vi "IB_RW_Project_MSI.vi"(7 "action":T1, 8 "error in (no error)":errorcluster, 9 "ProjectPath":path, 10 "MSI in":T2={"upgradeCode"="", "distID"="", "windowMessage"="", "windowTitle"="", "arpPhone"="", "arpContact"="", "arpURL"="http://", "arpCompany"="", "licenseID"="", "welcomeImageID"="", "bannerImageID"="", "osCheck"=0, "msiFileName"="", "cabFileName"="", "hwOption"=enum."<none>", "hwPath"=path "", "winsec.certificate"="", "winsec.timestamp"="", "winsec.description"="", "autoselect drivers"=FALSE, "hide non-runtimes"=FALSE}, 11 "Object In":T4) -> (0 "error out":errorcluster, 2 "MSI out":T2={"upgradeCode"="", "distID"="", "windowMessage"="", "windowTitle"="", "arpPhone"="", "arpContact"="", "arpURL"="http://", "arpCompany"="", "licenseID"="", "welcomeImageID"="", "bannerImageID"="", "osCheck"=0, "msiFileName"="", "cabFileName"="", "hwOption"=enum."<none>", "hwPath"=path "", "winsec.certificate"="", "winsec.timestamp"="", "winsec.description"="", "autoselect drivers"=FALSE, "hide non-runtimes"=FALSE}, 3 "Object Out":T4)   [LabVIEW 2020]
uses:
  <vilib>/AppBuilder/AB_Relative_Path_Type.ctl
  <resource>/Framework/Providers/API/ItemRef.ctl
  <resource>/Framework/Providers/Builds/Installer/CDK_sTypeDef_HWImportOption.ctl
  <vilib>/AppBuilder/IB_RW_Project/IB_RW_Project_MSI_Data.ctl
  <vilib>/AppBuilder/IB_RW_Project/IB_RW_Project_PropBag_Action.ctl
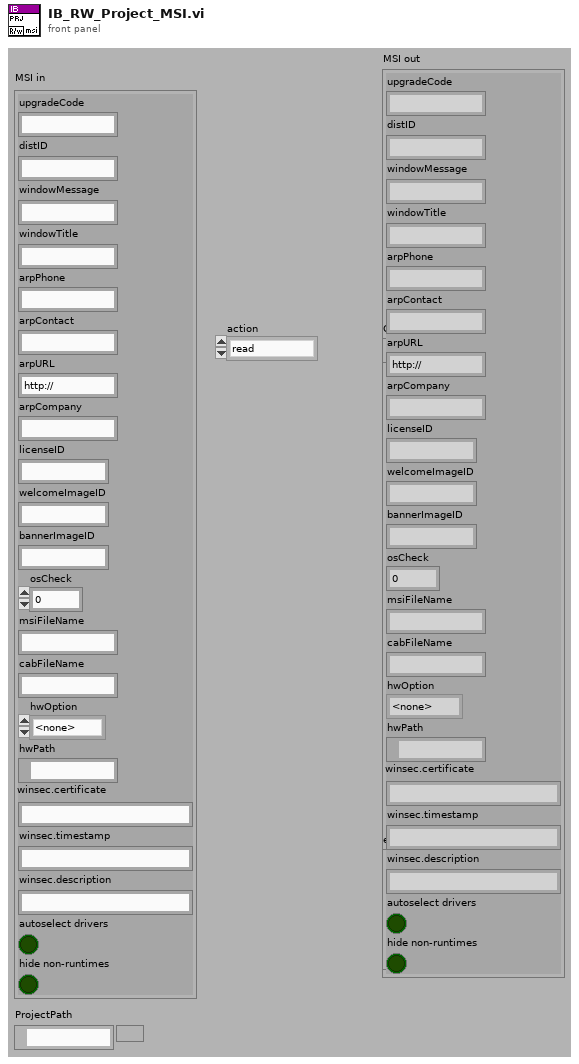
[diagram p1: front panel]
types:
  T1 = typedef "IB_RW_Project_PropBag_Action.ctl" = enum16{"read", "write", "clear", "readPrevious", "writePrevious", "clearPrevious"}
  T2 = typedef "IB_RW_Project_MSI_Data.ctl" = cluster{"upgradeCode":string, "distID":string, "windowMessage":string, "windowTitle":string, "arpPhone":string, "arpContact":string, "arpURL":string, "arpCompany":string, "licenseID":string, "welcomeImageID":string, "bannerImageID":string, "osCheck":i32, "msiFileName":string, "cabFileName":string, "hwOption":T3, "hwPath":path, "winsec.certificate":string, "winsec.timestamp":string, "winsec.description":string, "autoselect drivers":bool, "hide non-runtimes":bool}
  T3 = typedef "CDK_sTypeDef_HWImportOption.ctl" = enum16{"<none>", "Merge", "Replace", "Dialog"}
  T4 = typedef "ItemRef.ctl" = u64
  T5 = typedef "AB_Relative_Path_Type.ctl" = enum16{"<none>", "relativeToCommon", "relativeToAppDir", "relativeToProject"}
  T6 = typedef "IB_Relative_Path_Type.ctl" = enum16{"<none>", "relativeToCommon", "relativeToAppDir", "relativeToProject"}
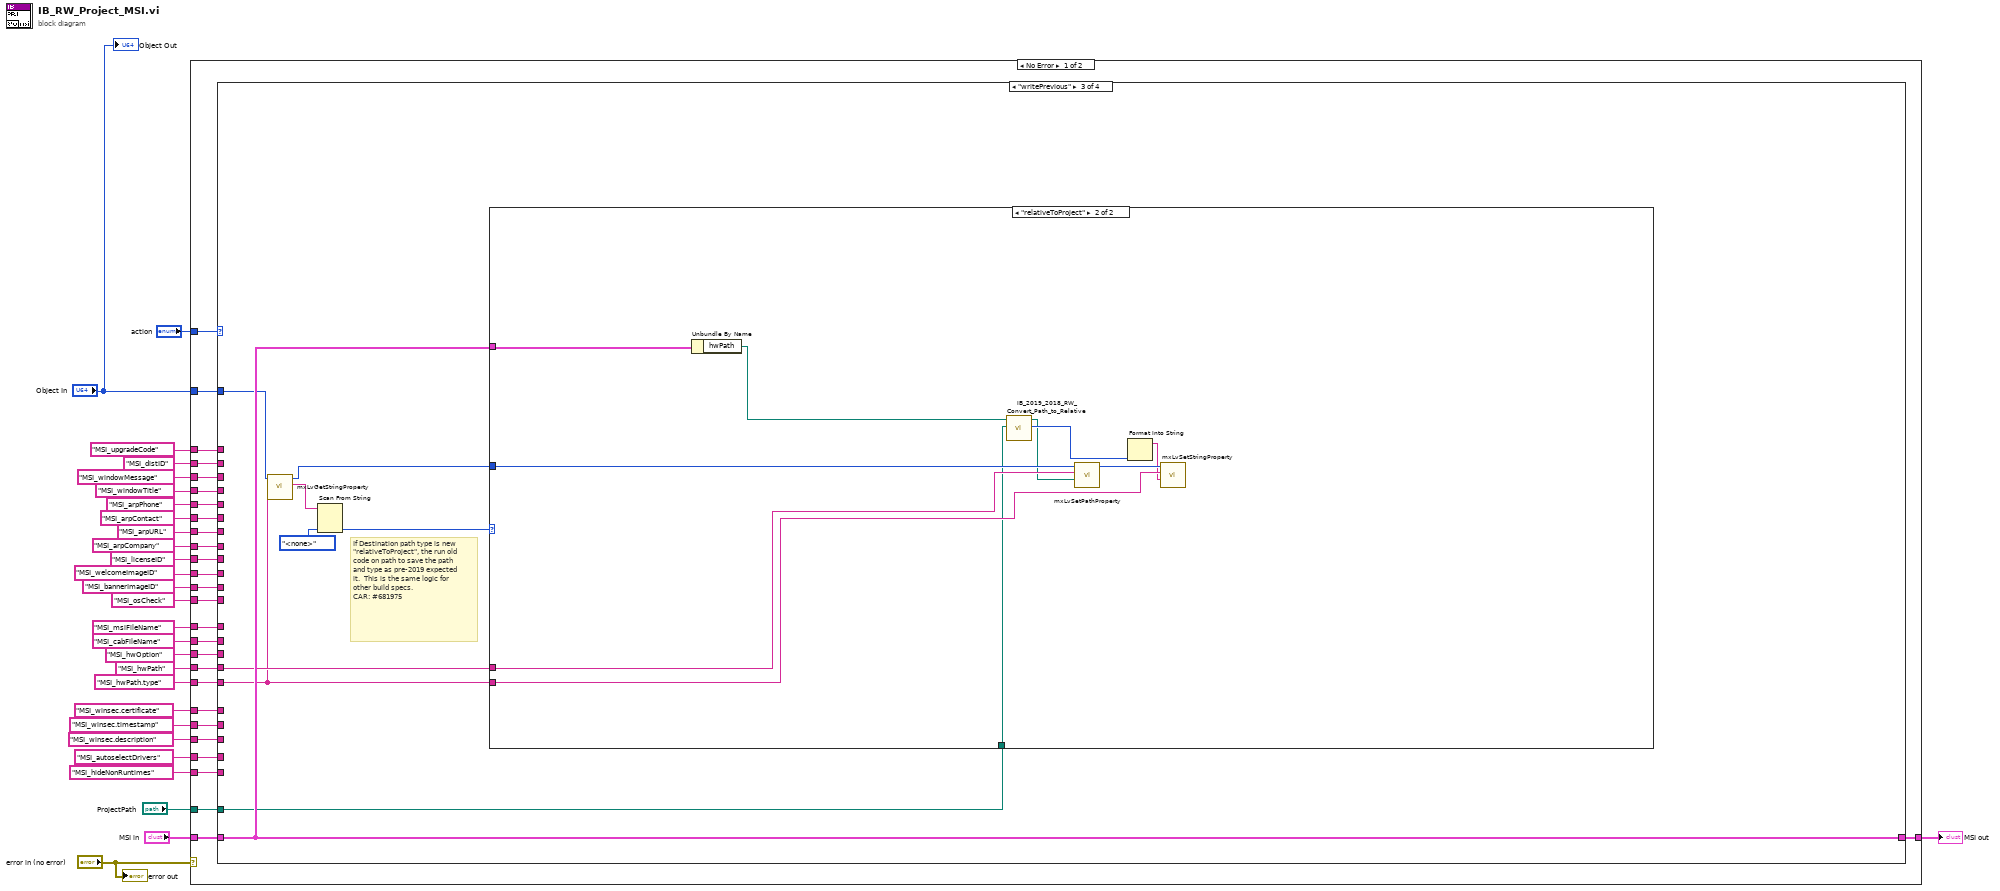
[diagram p0: block diagram]
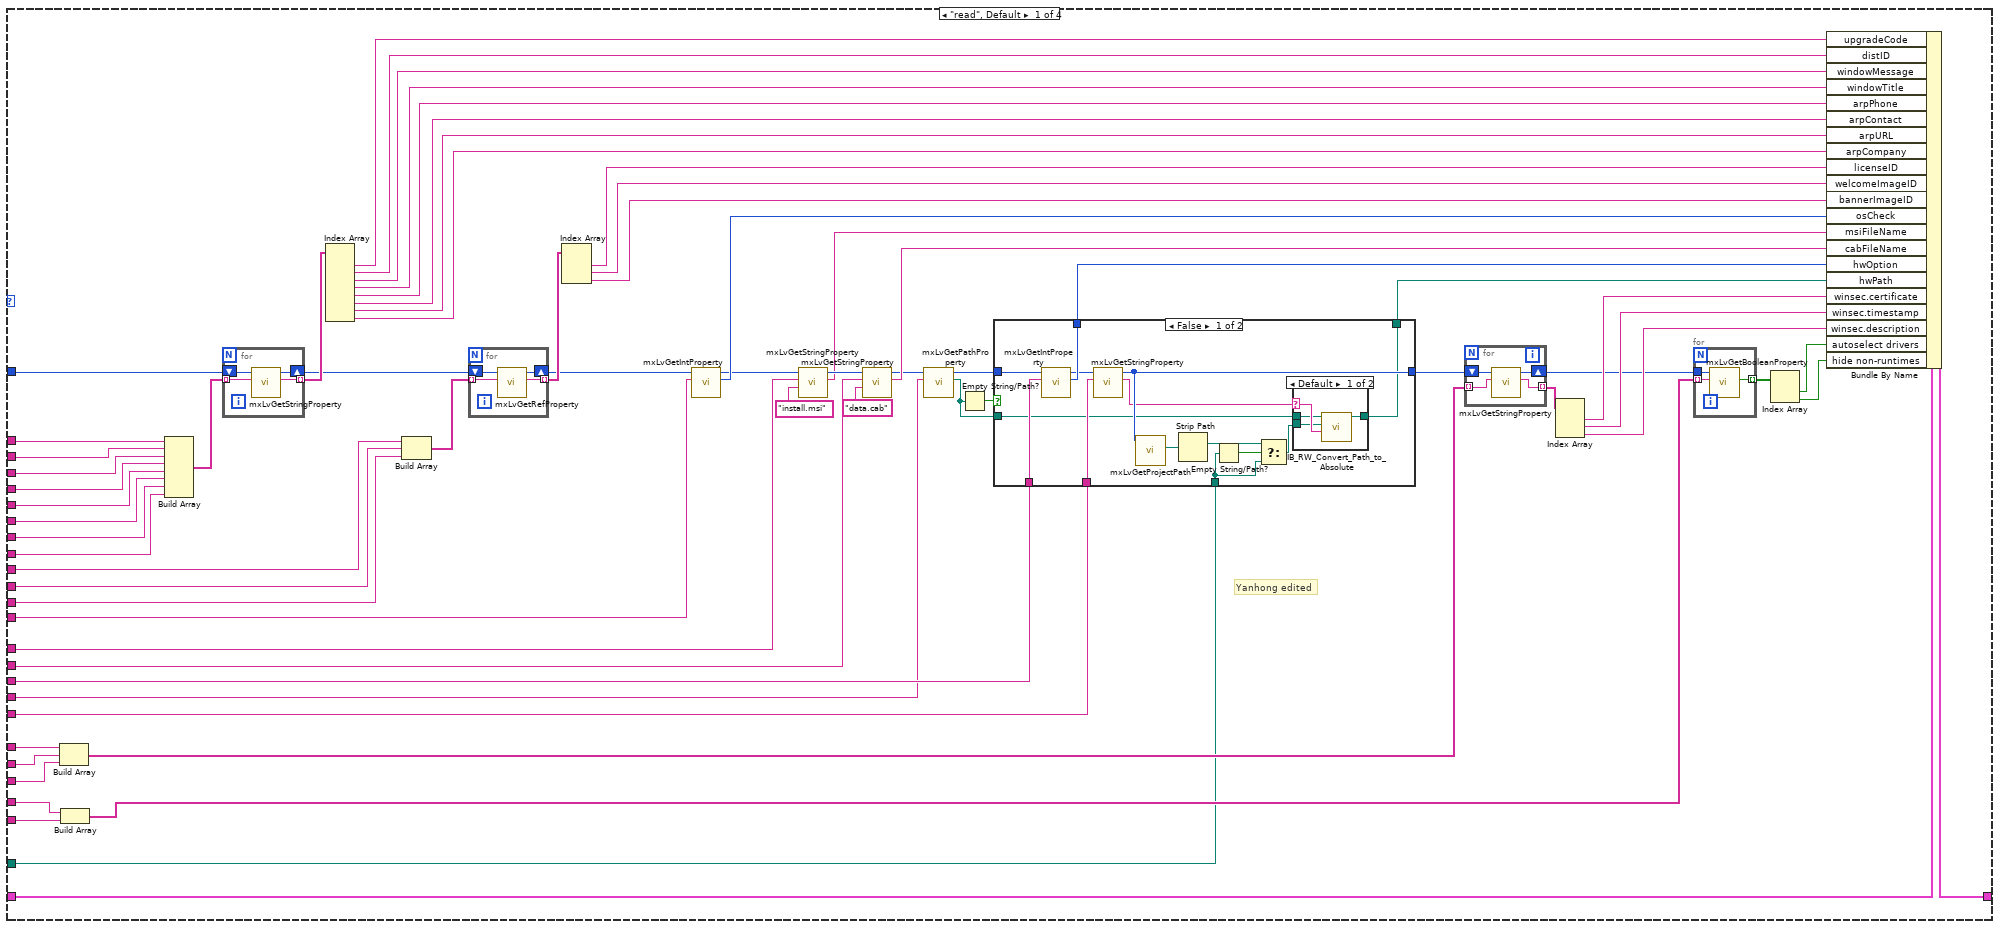
[diagram p2: hidden frame]
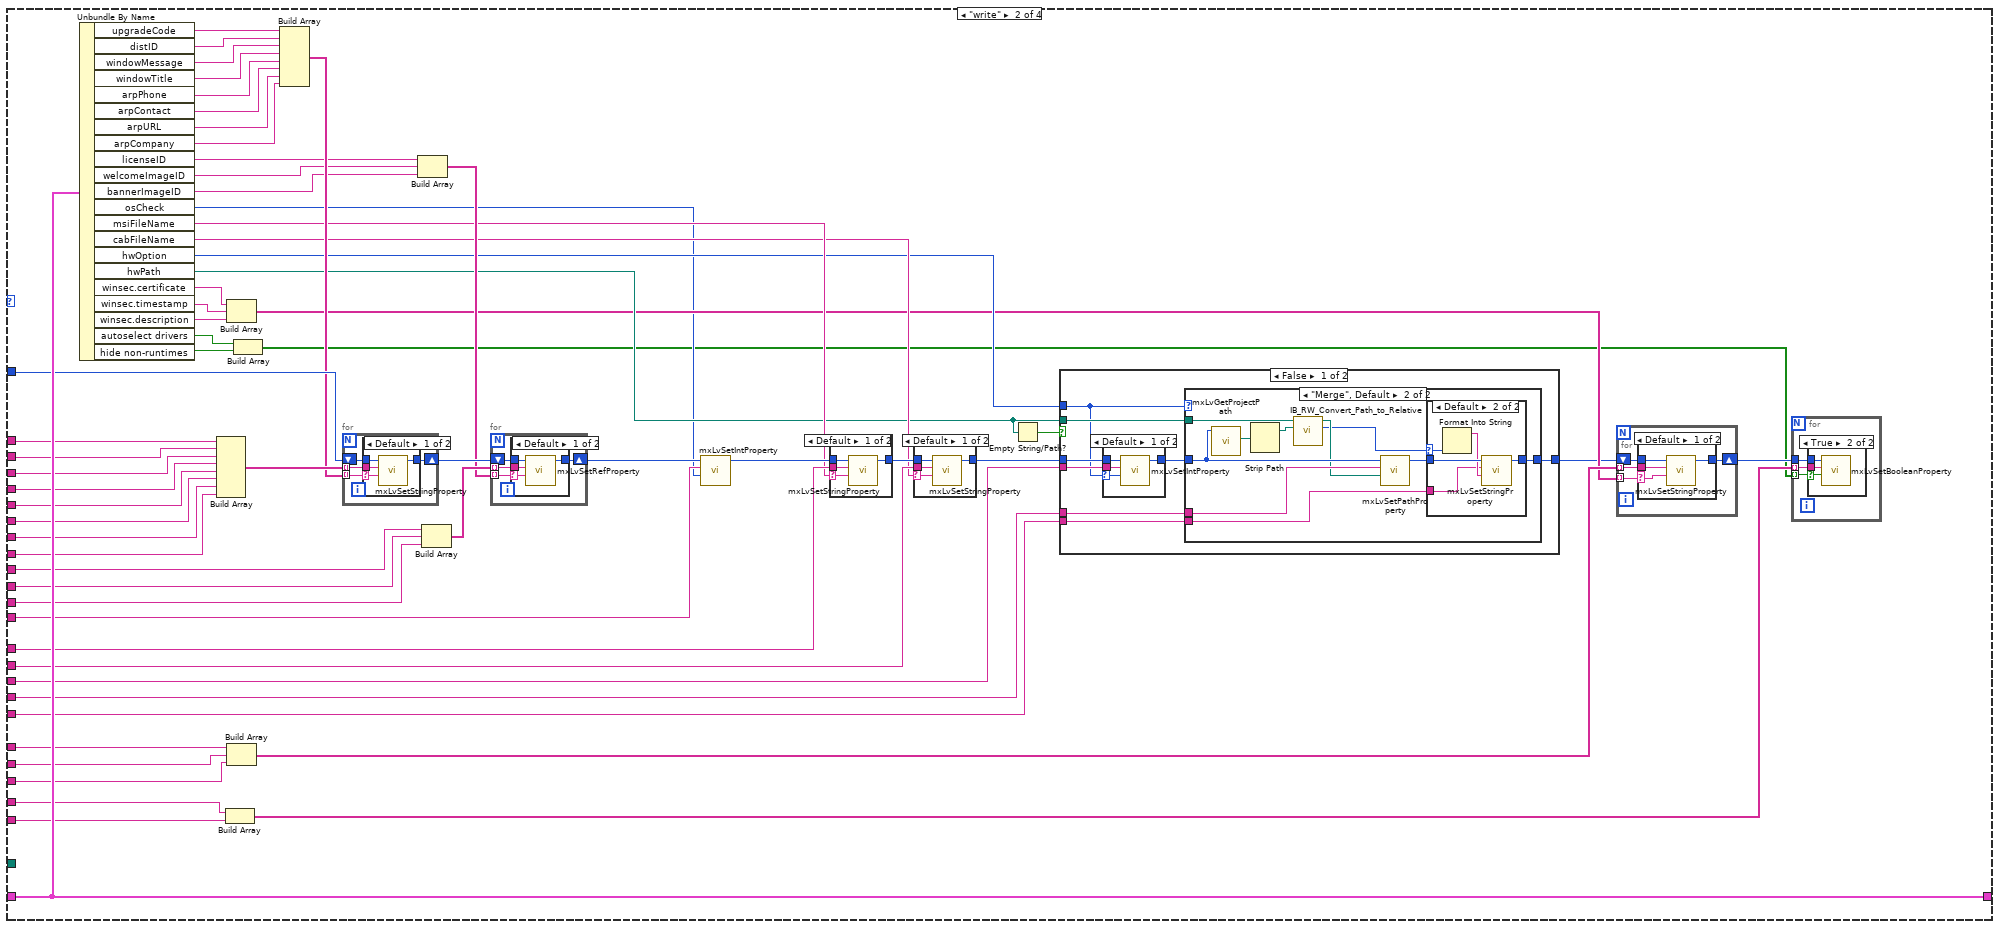
[diagram p5: hidden frame]
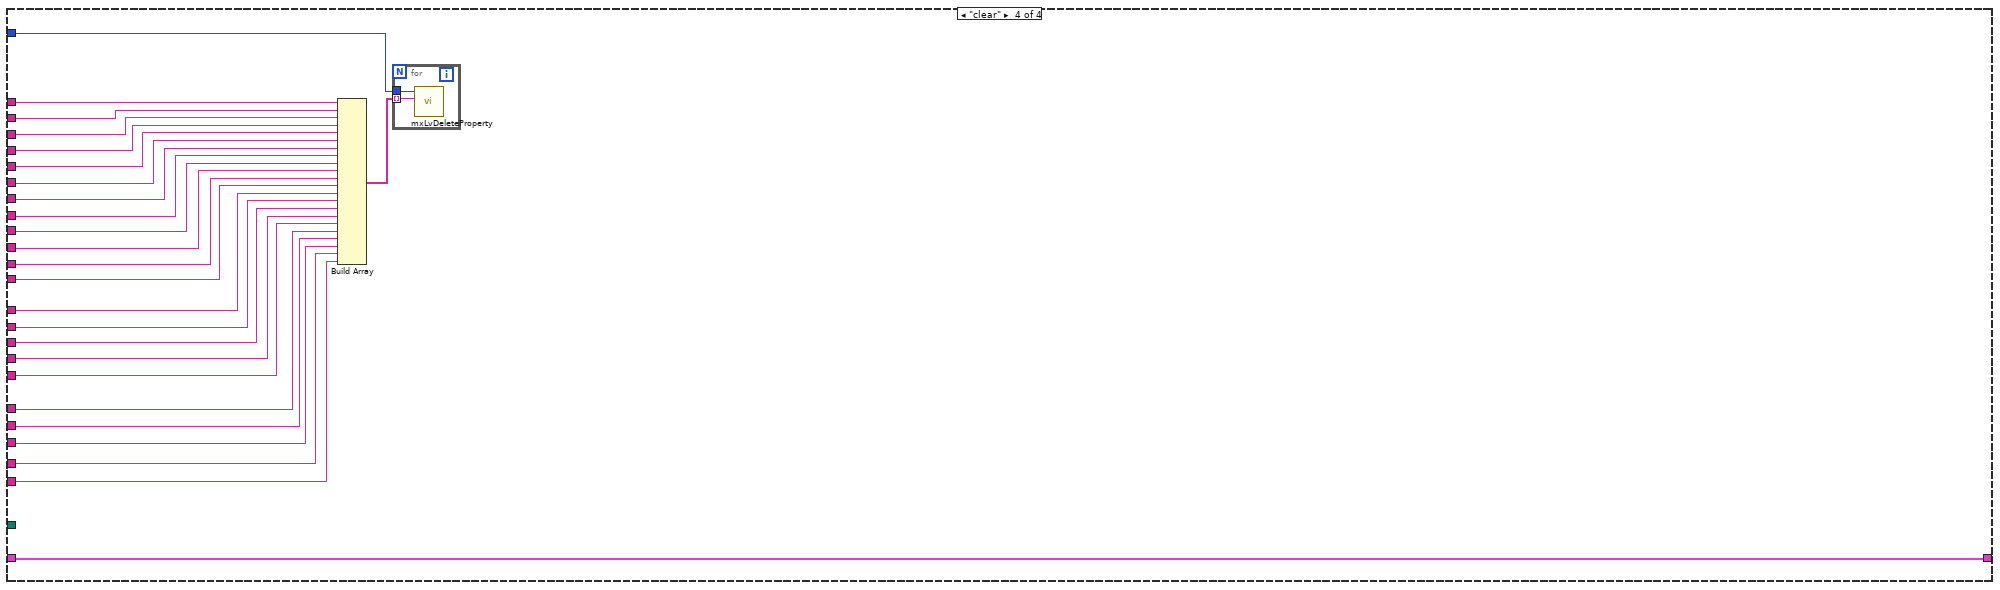
[diagram p17: hidden frame]
diagram:
  n1 = case shown="No Error" "error in (no error)" {
    tunnel: "Object In" -> [w55 _]
    tunnel: [w47 _] -> w26
    tunnel: "MSI_distID" ("Tag") -> [w52 _]
    tunnel: "MSI_windowMessage" ("Tag") -> [w51 _]
    tunnel: "MSI_arpURL" ("Tag") -> [w45 _]
    tunnel: "MSI_arpCompany" ("Tag") -> [w44 _]
    tunnel: "MSI_licenseID" ("Tag") -> [w43 _]
    tunnel: "MSI in" -> [w48 _]
    tunnel: "action" -> [w54 _]
    tunnel: "MSI_windowTitle" ("Tag") -> [w50 _]
    tunnel: "MSI_arpPhone" ("Tag") -> [w49 _]
    tunnel: "MSI_arpContact" ("Tag") -> [w46 _]
    tunnel: "MSI_upgradeCode" ("Tag") -> [w53 _]
    tunnel: "MSI_welcomeImageID" ("Tag") -> [w42 _]
    tunnel: "MSI_bannerImageID" ("Tag") -> [w41 _]
    tunnel: "MSI_osCheck" ("Tag") -> [w40 _]
    tunnel: "MSI_msiFileName" ("Tag") -> [w39 _]
    tunnel: "MSI_cabFileName" ("Tag") -> [w38 _]
    tunnel: "MSI_hwOption" ("Tag") -> [w37 _]
    tunnel: "MSI_hwPath" ("Tag") -> [w36 _]
    tunnel: "MSI_hwPath.type" ("Tag") -> [w35 _]
    tunnel: "MSI_winsec.certificate" ("Tag") -> [w34 _]
    tunnel: "MSI_winsec.timestamp" ("Tag") -> [w33 _]
    tunnel: "MSI_winsec.description" ("Tag") -> [w32 _]
    tunnel: "MSI_autoselectDrivers" ("Tag") -> [w31 _]
    tunnel: "MSI_hideNonRuntimes" ("Tag") -> [w30 _]
    tunnel: "ProjectPath" -> [w29 _]
    frame No Error {
      n2 = case shown="\"writePrevious\"" w54 {
        tunnel: [w122 w218 w301 w329] -> w47
        tunnel: w55 -> [w79 w217 w297 w336]
        tunnel: w48 -> [w121 w218 w301 w329]
        tunnel: w53 -> [w109 w216 _ w334]
        tunnel: w52 -> [w108 w215 _ w333]
        tunnel: w51 -> [w107 w214 _ w332]
        tunnel: w50 -> [w106 w213 _ w331]
        tunnel: w49 -> [w105 w212 _ w330]
        tunnel: w46 -> [w104 w211 _ w328]
        tunnel: w45 -> [w103 w210 _ w327]
        tunnel: w44 -> [w102 w209 _ w326]
        tunnel: w43 -> [w90 w197 _ w325]
        tunnel: w42 -> [w89 w196 _ w324]
        tunnel: w41 -> [w87 w195 _ w323]
        tunnel: w40 -> [w120 w168 _ w322]
        tunnel: w39 -> [w116 w188 _ w321]
        tunnel: w38 -> [w115 w185 _ w320]
        tunnel: w37 -> [w112 w177 _ w319]
        tunnel: w36 -> [w110 w182 w300 w318]
        tunnel: w35 -> [w80 w181 w296 w317]
        tunnel: w34 -> [w74 w173 _ w316]
        tunnel: w33 -> [w73 w172 _ w315]
        tunnel: w32 -> [w72 w171 _ w314]
        tunnel: w31 -> [w61 w162 _ w313]
        tunnel: w30 -> [w62 w163 _ w312]
        tunnel: w29 -> [w56 _ w293 _]
        frame "read", Default {
          # "Yanhong edited"
          n3 = Build Array(w74, w73, w72) -> (w71:string[])
          n4 = Build Array(w61, w62) -> (w60:string[])
          n5 = Build Array(w109, w108, w107, w106, w105, w104, w103, w102) -> (w101:string[])
          n6 = for {
            tunnel: [w157] -> w100 mode=indexing
            tunnel: w101 -> [w156] mode=indexing
            shift-right: [w154] -> w91
            shift-left: w79 -> [w155]
            n7 = call <resource>:"mxLvGetStringProperty.vi"("Tag"=w156, "Item"=w155) -> ("Value"=w157:string, "Item"=w154:T4)  [unwired: 1 in, 7 out]
          }
          n8 = Index Array(array=w100) -> (element #1=w99:string, element #2=w98:string, element #3=w97:string, element #4=w96:string, element #5=w95:string, element #6=w94:string, element #7=w93:string, element #8=w92:string)  [unwired: 8 in]
          n9 = Build Array(w90, w89, w87) -> (w88:string[])
          n10 = for {
            shift-right: [w152] -> w82
            shift-left: w91 -> [w153]
            tunnel: w88 -> [w151] mode=indexing
            tunnel: [w150] -> w86 mode=indexing
            n11 = call <resource>:"mxLvGetRefProperty.vi"("Tag"=w151, "Item"=w153) -> ("Value"=w150:string, "Item"=w152:T4)  [unwired: 1 in, 7 out]
          }
          n12 = Index Array(array=w86) -> (element #1=w85:string, element #2=w84:string, element #3=w83:string)  [unwired: 3 in]
          n13 = call <resource>:"mxLvGetIntProperty.vi"("Tag"=w120, "Item"=w82) -> ("Value"=w66:i32, "Item"=w65:T4)  [unwired: 1 in, 7 out]
          n14 = call <resource>:"mxLvGetStringProperty.vi"("Default Value (\"\")"="install.msi", "Tag"=w116, "Item"=w65) -> ("Value"=w114:string, "Item"=w117:T4)  [unwired: 1 in, 6 out]
          n15 = call <resource>:"mxLvGetStringProperty.vi"("Default Value (\"\")"="data.cab", "Tag"=w115, "Item"=w117) -> ("Value"=w113:string, "Item"=w78:T4)  [unwired: 1 in, 6 out]
          n16 = call <resource>:"mxLvGetPathProperty.vi"("Tag"=w110, "Item"=w78) -> ("Path"=w76:path, "Item"=w77:T4)  [unwired: 2 in, 6 out]
          n17 = Empty String/Path?(string/path=w76) -> (empty?=w75:bool)
          n18 = case shown="False" w75 {
            tunnel: w112 -> [w143 _]
            tunnel: [w142 _] -> w111
            tunnel: [w135 _] -> w81
            tunnel: w76 -> [w136 _]
            tunnel: w80 -> [w140 _]
            tunnel: w77 -> [w139 w149]
            tunnel: [w137 w149] -> w64
            tunnel: w56 -> [w130 _]
            frame False {
              n19 = call <resource>:"mxLvGetIntProperty.vi"("Tag"=w143, "Item"=w139) -> ("Value"=w142:i32, "Item"=w138:T4)  [unwired: 1 in, 7 out]
              n20 = call <resource>:"mxLvGetStringProperty.vi"("Tag"=w140, "Item"=w138) -> ("Value"=w134:string, "Item"=w137:T4)  [unwired: 1 in, 7 out]
              n21 = call <resource>:"mxLvGetProjectPath.vi"("Item"=w137) -> ("Project Path"=w141:path)  [unwired: 1 in, 9 out]
              n22 = Strip Path(path=w141) -> (stripped path=w131:path)  [unwired: 1 out]
              n23 = Empty String/Path?(string/path=w130) -> (empty?=w133:bool)
              n24 = Select(t=w131, s=w133, f=w130) -> (s? t:f=w132:path)
              n25 = case shown="Default" w134 {
                selector: w134 -> [w147 _]
                tunnel: [w146 w148] -> w135
                tunnel: w136 -> [w145 w148]
                tunnel: w132 -> [w144 _]
                frame Default {
                  n26 = call <vilib>:"IB_RW_Convert_Path_to_Absolute.vi"("relativeType"=w147, "commonPath"=w144, "relativePath"=w145) -> ("absolute path"=w146:path)  [unwired: 7 in, 1 out]
                }
                frame "" {
                }
              }
            }
            frame True {
            }
          }
          n27 = for {
            shift-right: [w128] -> w63
            shift-left: w64 -> [w129]
            tunnel: w71 -> [w126] mode=indexing
            tunnel: [w127] -> w70 mode=indexing
            n28 = call <resource>:"mxLvGetStringProperty.vi"("Tag"=w126, "Item"=w129) -> ("Value"=w127:string, "Item"=w128:T4)  [unwired: 1 in, 7 out]
          }
          n29 = Index Array(array=w70) -> (element #1=w69:string, element #2=w68:string, element #3=w67:string)  [unwired: 3 in]
          n30 = for {
            tunnel: w63 -> [w125]
            tunnel: [w124] -> w59 mode=indexing
            tunnel: w60 -> [w123] mode=indexing
            n31 = call <resource>:"mxLvGetBooleanProperty.vi"("Tag"=w123, "Item"=w125) -> ("Value"=w124:bool)  [unwired: 2 in, 7 out]
          }
          n32 = Index Array(array=w59) -> (element #1=w58:bool, element #2=w57:bool)  [unwired: 2 in]
          n33 = Bundle By Name(cluster=w121, "upgradeCode"=w99, "distID"=w98, "windowMessage"=w97, "windowTitle"=w96, "arpPhone"=w95, "arpContact"=w94, "arpURL"=w93, "arpCompany"=w92, "licenseID"=w85, "welcomeImageID"=w84, "bannerImageID"=w83, "osCheck"=w66, "msiFileName"=w114, "cabFileName"=w113, "hwOption"=w111, "hwPath"=w81, "winsec.certificate"=w69, "winsec.timestamp"=w68, "winsec.description"=w67, "autoselect drivers"=w58, "hide non-runtimes"=w57) -> (w122:T2)
        }
        frame "write" {
          n34 = Unbundle By Name(w218) -> ("upgradeCode"=w207:string, "distID"=w206:string, "windowMessage"=w205:string, "windowTitle"=w204:string, "arpPhone"=w203:string, "arpContact"=w202:string, "arpURL"=w201:string, "arpCompany"=w200:string, "licenseID"=w193:string, "welcomeImageID"=w192:string, "bannerImageID"=w191:string, "osCheck"=w166:i32, "msiFileName"=w187:string, "cabFileName"=w184:string, "hwOption"=w183:T3, "hwPath"=w180:path, "winsec.certificate"=w176:string, "winsec.timestamp"=w175:string, "winsec.description"=w174:string, "autoselect drivers"=w159:bool, "hide non-runtimes"=w160:bool)
          n35 = Build Array(w216, w215, w214, w213, w212, w211, w210, w209) -> (w208:string[])
          n36 = Build Array(w162, w163) -> (w161:string[])
          n37 = Build Array(w176, w175, w174) -> (w169:string[])
          n38 = Build Array(w173, w172, w171) -> (w170:string[])
          n39 = Build Array(w159, w160) -> (w158:bool[])
          n40 = Build Array(w207, w206, w205, w204, w203, w202, w201, w200) -> (w199:string[])
          n41 = for {
            shift-right: [w287] -> w198
            shift-left: w217 -> [w286]
            tunnel: w208 -> [w285] mode=indexing
            tunnel: w199 -> [w284] mode=indexing
            n42 = case shown="Default" w284 {
              selector: w284 -> [w289 _]
              tunnel: w286 -> [w291 w292]
              tunnel: [w290 w292] -> w287
              tunnel: w285 -> [w288 _]
              frame Default {
                n43 = call <resource>:"mxLvSetStringProperty.vi"("Value (\"\")"=w289, "Tag"=w288, "Item"=w291) -> ("Item"=w290:T4)  [unwired: 2 in, 6 out]
              }
              frame "" {
              }
            }
          }
          n44 = Build Array(w193, w192, w191) -> (w190:string[])
          n45 = Build Array(w197, w196, w195) -> (w194:string[])
          n46 = for {
            shift-right: [w278] -> w167
            shift-left: w198 -> [w277]
            tunnel: w194 -> [w276] mode=indexing
            tunnel: w190 -> [w275] mode=indexing
            n47 = case shown="Default" w275 {
              selector: w275 -> [w280 _]
              tunnel: w277 -> [w279 w283]
              tunnel: [w282 w283] -> w278
              tunnel: w276 -> [w281 _]
              frame Default {
                n48 = call <resource>:"mxLvSetRefProperty.vi"("Value (\"\")"=w280, "Tag"=w281, "Item"=w279) -> ("Item"=w282:T4)  [unwired: 2 in, 6 out]
              }
              frame "" {
              }
            }
          }
          n49 = call <resource>:"mxLvSetIntProperty.vi"("Value (0)"=w166, "Tag"=w168, "Item"=w167) -> ("Item"=w189:T4)  [unwired: 2 in, 6 out]
          n50 = case shown="Default" w187 {
            selector: w187 -> [w271 _]
            tunnel: w189 -> [w273 w274]
            tunnel: w188 -> [w272 _]
            tunnel: [w270 w274] -> w186
            frame Default {
              n51 = call <resource>:"mxLvSetStringProperty.vi"("Value (\"\")"=w271, "Tag"=w272, "Item"=w273) -> ("Item"=w270:T4)  [unwired: 2 in, 6 out]
            }
            frame "install.msi" {
            }
          }
          n52 = case shown="Default" w184 {
            selector: w184 -> [w266 _]
            tunnel: w186 -> [w268 w269]
            tunnel: w185 -> [w267 _]
            tunnel: [w265 w269] -> w178
            frame Default {
              n53 = call <resource>:"mxLvSetStringProperty.vi"("Value (\"\")"=w266, "Tag"=w267, "Item"=w268) -> ("Item"=w265:T4)  [unwired: 2 in, 6 out]
            }
            frame "data.cab" {
            }
          }
          n54 = Empty String/Path?(string/path=w180) -> (empty?=w179:bool)
          n55 = case shown="False" w179 {
            tunnel: w178 -> [w237 w264]
            tunnel: w183 -> [w234 _]
            tunnel: w182 -> [w241 _]
            tunnel: w180 -> [w240 _]
            tunnel: [w239 w264] -> w165
            tunnel: w181 -> [w238 _]
            tunnel: w177 -> [w235 _]
            frame False {
              n56 = case shown="Default" w234 {
                selector: w234 -> [w243 _]
                tunnel: w237 -> [w245 w246]
                tunnel: w235 -> [w244 _]
                tunnel: [w242 w246] -> w236
                frame Default {
                  n57 = call <resource>:"mxLvSetIntProperty.vi"("Value (0)"=w243, "Tag"=w244, "Item"=w245) -> ("Item"=w242:T4)  [unwired: 2 in, 6 out]
                }
                frame "<none>" {
                }
              }
              n58 = case shown="\"Merge\", Default" w234 {
                tunnel: w236 -> [w247 w252]
                tunnel: w241 -> [_ w257]
                tunnel: w240 -> [_ w250]
                tunnel: w238 -> [_ w255]
                tunnel: [w247 w248] -> w239
                frame "<none>" {
                }
                frame "Merge", Default {
                  n59 = call <resource>:"mxLvGetProjectPath.vi"("Item"=w252) -> ("Project Path"=w253:path)  [unwired: 1 in, 9 out]
                  n60 = Strip Path(path=w253) -> (stripped path=w254:path)  [unwired: 1 out]
                  n61 = call <vilib>:"IB_RW_Convert_Path_to_Relative.vi"("commonPath"=w254, "absolutePath"=w250) -> ("relativeType"=w249:T5, "newPath"=w251:path)  [unwired: 7 in, 1 out]
                  n62 = call <resource>:"mxLvSetPathProperty.vi"("Path"=w251, "Tag"=w257, "Item"=w252) -> ("Item"=w256:T4)  [unwired: 2 in, 6 out]
                  n63 = case shown="Default" w249 {
                    selector: w249 -> [_ w260]
                    tunnel: w256 -> [w258 w263]
                    tunnel: w255 -> [_ w261]
                    tunnel: [w258 w259] -> w248
                    frame "<none>" {
                    }
                    frame Default {
                      n64 = Format Into String(w260) -> (resulting string=w262:string)  [unwired: 3 in, 1 out]
                      n65 = call <resource>:"mxLvSetStringProperty.vi"("Value (\"\")"=w262, "Tag"=w261, "Item"=w263) -> ("Item"=w259:T4)  [unwired: 2 in, 6 out]
                    }
                  }
                }
              }
            }
            frame True {
            }
          }
          n66 = for {
            tunnel: w169 -> [w227] mode=indexing
            shift-right: [w226] -> w164
            shift-left: w165 -> [w228]
            tunnel: w170 -> [w225] mode=indexing
            n67 = case shown="Default" w227 {
              selector: w227 -> [w230 _]
              tunnel: w228 -> [w232 w233]
              tunnel: w225 -> [w229 _]
              tunnel: [w231 w233] -> w226
              frame Default {
                n68 = call <resource>:"mxLvSetStringProperty.vi"("Value (\"\")"=w230, "Tag"=w229, "Item"=w232) -> ("Item"=w231:T4)  [unwired: 2 in, 6 out]
              }
              frame "" {
              }
            }
          }
          n69 = for {
            tunnel: w164 -> [w221]
            tunnel: w158 -> [w220] mode=indexing
            tunnel: w161 -> [w219] mode=indexing
            n70 = case shown="True" w220 {
              selector: w220 -> [_ w222]
              tunnel: w221 -> [_ w224]
              tunnel: w219 -> [_ w223]
              frame False {
              }
              frame True {
                n71 = call <resource>:"mxLvSetBooleanProperty.vi"("Value (F)"=w222, "Tag"=w223, "Item"=w224) -> ()  [unwired: 2 in, 7 out]
              }
            }
          }
        }
        frame "writePrevious" {
          # "If Destination path type is new \"relativeToProject\", the run old code on path to save the path and type as pre-2019 expected it.  This is the same logic for other build specs.\nCAR: #681975"
          n72 = call <resource>:"mxLvGetStringProperty.vi"("Tag"=w296, "Item"=w297) -> ("Value"=w299:string, "Item"=w294:T4)  [unwired: 1 in, 7 out]
          n73 = Scan From String(input string=w299, default 1=AB_Relative_Path_Type."<none>" ("relativeType")) -> (output 1=w295:T5)  [unwired: 3 in, 3 out]
          n74 = case shown="\"relativeToProject\"" w295 {
            tunnel: w301 -> [_ w311]
            tunnel: w294 -> [_ w310]
            tunnel: w300 -> [_ w309]
            tunnel: w296 -> [_ w308]
            tunnel: w293 -> [_ w302]
            frame Default {
            }
            frame "relativeToProject" {
              n75 = Unbundle By Name(w311) -> ("hwPath"=w305:path)
              n76 = call <vilib>:"IB_2019_2018_RW_Convert_Path_to_Relative.vi"("commonPath"=w302, "absolutePath"=w305) -> ("relativeType"=w304:T6, "newPath"=w303:path)  [unwired: 7 in, 1 out]
              n77 = call <resource>:"mxLvSetPathProperty.vi"("Path"=w303, "Tag"=w309, "Item"=w310) -> ("Item"=w307:T4)  [unwired: 2 in, 6 out]
              n78 = Format Into String(w304) -> (resulting string=w306:string)  [unwired: 3 in, 1 out]
              n79 = call <resource>:"mxLvSetStringProperty.vi"("Value (\"\")"=w306, "Tag"=w308, "Item"=w307) -> ()  [unwired: 2 in, 7 out]
            }
          }
        }
        frame "clear" {
          n80 = Build Array(w334, w333, w332, w331, w330, w328, w327, w326, w325, w324, w323, w322, w321, w320, w319, w318, w317, w316, w315, w314, w313, w312) -> (w335:string[])
          n81 = for {
            tunnel: w336 -> [w338]
            tunnel: w335 -> [w337] mode=indexing
            n82 = call <resource>:"mxLvDeleteProperty.vi"("Tag"=w337, "Item"=w338) -> ()  [unwired: 1 in, 9 out]
          }
        }
      }
    }
    frame Error {
    }
  }
  "MSI out" <- w26
  "Object Out" <- "Object In"
  "error out" <- "error in (no error)"
